vi "Auto Detect_Programming Mode_Initialize UI Elements.vi"(8 "error in":errorcluster, 10 "References":refnum<vi>[](array[refnum]), 11 "NumSlots":i32) -> (0 "error out":errorcluster, 1 "Programming Mode Out":T1[](array[typedef]))   [LabVIEW 2017, in "Scan Engine Custom Device.lvlib"]
doc: "Initialize Slot Programming Modes Controls (8 elements). We use individual elements because we want to be able to control respective \"Enable State\"."
uses:
  Scan Engine Custom Device.lvlib
  Type Defs/Slot - Slot Programming Mode.ctl
  Type Defs/Slot Programming Mode.ctl
panel:
  in  "Slot Programming Mode":T1
  in  "Slot 2":string
  in  "Slot":T2
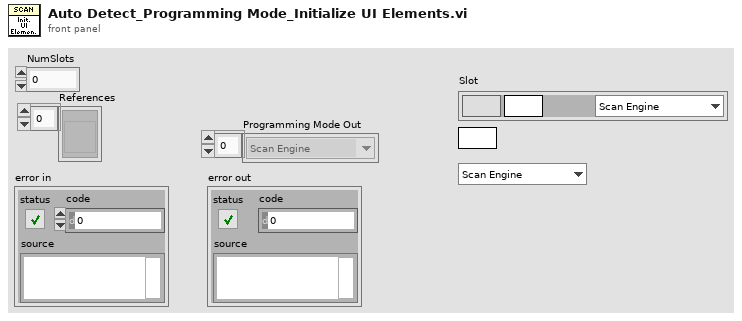
[diagram p1: front panel]
types:
  T1 = typedef "Scan Engine Custom Device.lvlib/Slot Programming Mode.ctl" = enum16{"Scan Engine", "LabVIEW FPGA", "NI-DAQmx", "Don't Modify"}
  T2 = typedef "Slot - Slot Programming Mode.ctl" = cluster{"Slot":string, "Module Name":string, "Slot Programming Mode":enum16{"Scan Engine", "LabVIEW FPGA", "NI-DAQmx", "Don't Modify"}}
  T3 = enum8{"Enabled", "Disabled", "Disabled and Grayed Out"}
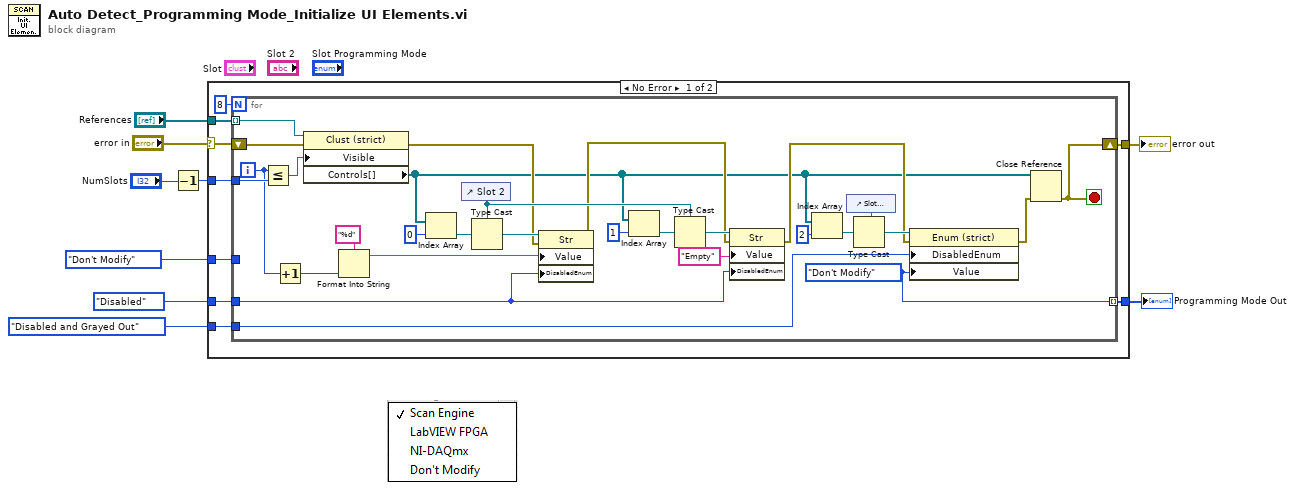
[diagram p0: block diagram]
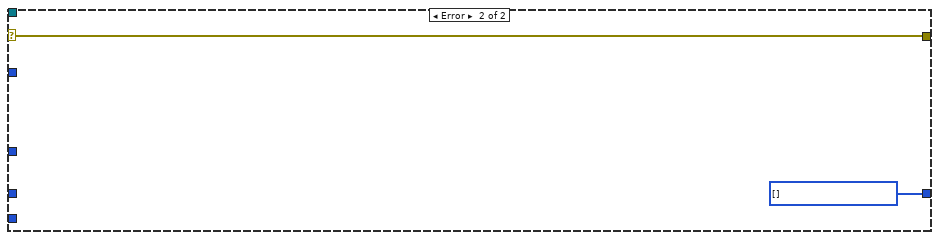
[diagram p2: hidden frame]
diagram:
  n1 = Decrement(x="NumSlots") -> (x-1=w3:i32)
  n2 = case shown="No Error" "error in" {
    selector: "error in" -> [w15 w49]
    tunnel: "References" -> [w18 _]
    tunnel: T3."Disabled" ("Disabled") -> [w17 _]
    tunnel: [w16 w49] -> w7
    tunnel: Slot_Programming_Mode."Don't Modify" ("Value") -> [w14 _]
    tunnel: w3 -> [w12 _]
    tunnel: T3."Disabled and Grayed Out" ("Disabled") -> [w11 _]
    tunnel: [w10 w48] -> w1
    frame No Error {
      n3 = for {
        N: 8 -> [_]
        tunnel: w18 -> [w46] mode=indexing
        shift-right: [w21] -> w16
        shift-left: w15 -> [w45]
        tunnel: w17 -> [w32]
        tunnel: w14 -> [_]
        tunnel: w12 -> [w47]
        tunnel: w11 -> [w27]
        tunnel: [w26] -> w10 mode=indexing
        i -> [w41]
        stop <- w21 stop-if-true
        w26 = Slot_Programming_Mode."Don't Modify" ("Value")
        n4 = Less Or Equal?(x=w41, y=w47) -> (x <= y?=w19:bool)
        n5 = Increment(x=w41) -> (x+1=w40:i32)
        n6 = property class="Clust (strict)"(reference=w46, error in=w45, "Visible"=w19) -> (error out=w25:errorcluster, "Controls[]"=w20:refnum<vi>[])  [unwired: 1 out]
        n7 = Format Into String(format string="%d", w40) -> (resulting string=w38:string)  [unwired: 2 in, 1 out]
        n8 = Index Array(array=w20, index=0) -> (element=w43:refnum<vi>)
        n9 = control-ref of="Slot 2"() -> (w34:refnum<vi>)
        n10 = Type Cast(type=w34, x=w43) -> (*(type *) &x=w42:refnum<vi>)
        n11 = property class="Str"(reference=w42, error in=w25, "Value"=w38, "DisabledEnum"=w32) -> (error out=w24:errorcluster)  [unwired: 1 out]
        n12 = Index Array(array=w20, index=1) -> (element=w36:refnum<vi>)
        n13 = Type Cast(type=w34, x=w36) -> (*(type *) &x=w37:refnum<vi>)
        n14 = property class="Str"(reference=w37, error in=w24, "Value"="Empty", "DisabledEnum"=w32) -> (error out=w22:errorcluster)  [unwired: 1 out]
        n15 = Index Array(array=w20, index=2) -> (element=w29:refnum<vi>)
        n16 = control-ref of="Slot Programming Mode"() -> (w30:refnum<vi>)
        n17 = Type Cast(type=w30, x=w29) -> (*(type *) &x=w28:refnum<vi>)
        n18 = property class="Enum (strict)"(reference=w28, error in=w22, "DisabledEnum"=w27, "Value"=w26) -> (error out=w23:errorcluster)  [unwired: 1 out]
        n19 = Close Reference(reference=w20, error in (no error)=w23) -> (error out=w21:errorcluster)
      }
    }
    frame Error {
      w48 = T1[] [] items=["Scan Engine", "LabVIEW FPGA", "NI-DAQmx", "Don't Modify"]
    }
  }
  "error out" <- w7
  "Programming Mode Out" <- w1
